vi "domeADB_getEvent_RotationPrevented.vi"(8 "error in (no error)":errorcluster, 11 "logevent_RotationPrevented_Ctl":T1) -> (0 "error out":errorcluster, 2 "function return":i32, 3 "logevent_RotationPrevented_Ctl out":T1)   [LabVIEW 2015, in "SALLV_domeADB.lvlib"]
doc: "int domeADB_shm_getEvent_RotationPreventedLV(domeADB_logevent_RotationPreventedLV *logevent_RotationPrevented_Ctl );"
uses:
  SALLV_domeADB.lvlib
  DataTypes/logevent_RotationPrevented.ctl
  SALLV_domeADB.so
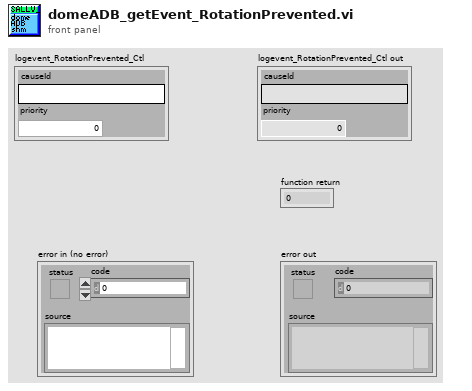
[diagram p1: front panel]
types:
  T1 = typedef "SALLV_domeADB.lvlib/logevent_RotationPrevented.ctl" = cluster{"causeId":string, "priority":i32}
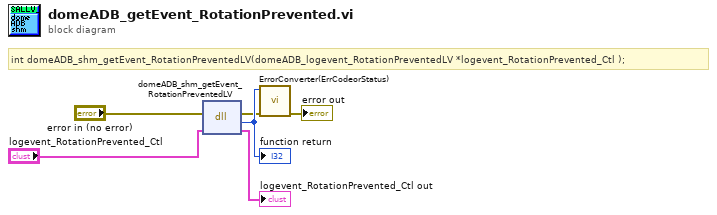
[diagram p0: block diagram]
diagram:
  # "int domeADB_shm_getEvent_RotationPreventedLV(domeADB_logevent_RotationPreventedLV *logevent_RotationPrevented_Ctl );"
  n1 = dll-call lib="home/andres/Desktop/SALLV_domeADB2015/SALLV_domeADB.*" fn="domeADB_shm_getEvent_RotationPreventedLV"(error in="error in (no error)", "logevent_RotationPrevented_Ctl"="logevent_RotationPrevented_Ctl") -> (error out=w2:errorcluster, w6:i32, "logevent_RotationPrevented_Ctl"=→"logevent_RotationPrevented_Ctl out":T1)  [unwired: 2 in, 1 out]
  "function return" <- w6
  n2 = call "ErrorConverter(ErrCodeorStatus).vi"("error in (no error)"=w2, "error code"=w6) -> ("error out"=→"error out":errorcluster)  [unwired: 9 in]
